vi "Create Cluster BasedOn Item.vi"(10 "Item Value":variant, 11 "Item Type":T1) -> (3 "Cluster":cluster{"Type":T1, "Value":variant})   [LabVIEW 2024, in "Config File Parser.lvlib"]
uses:
  Config File Parser.lvlib
  Item/Item Type.ctl
  Item/Item.lvclass
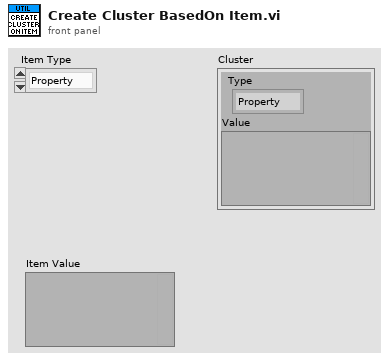
[diagram p1: front panel]
types:
  T1 = typedef "Config File Parser.lvlib/Item.lvclass/Item Type.ctl" = enum16{"Property", "Channel", "Section"}
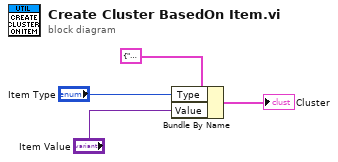
[diagram p0: block diagram]
diagram:
  n1 = Bundle By Name(cluster=cluster{"Type":T1, "Value":variant} {"Type"=enum."Property", "Value"=variant}, "Type"="Item Type", "Value"="Item Value") -> (→"Cluster":cluster{"Type":T1, "Value":variant})
